vi "Xsens DeltaV (SubVI).vi"(1 "DATA in (Hex)":string) -> (0 "DeltaV":T1 {"DeltaVZ (m/s)" format="%#.7f"})   [LabVIEW 2019]
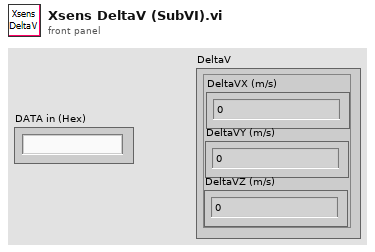
[diagram p1: front panel]
types:
  T1 = cluster{"DeltaVX (m/s)":sgl, "DeltaVY (m/s)":sgl, "DeltaVZ (m/s)":sgl}
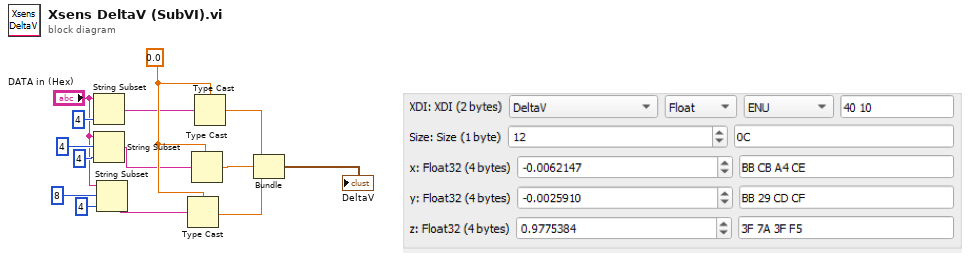
[diagram p0: block diagram]
diagram:
  w10 = sgl 0.0
  n1 = String Subset(string="DATA in (Hex)", length (rest)=4 ("length (rest)")) -> (substring=w8:string)  [unwired: 1 in]
  n2 = String Subset(string="DATA in (Hex)", offset (0)=4, length (rest)=4 ("length (rest)")) -> (substring=w3:string)
  n3 = String Subset(string="DATA in (Hex)", offset (0)=8, length (rest)=4 ("length (rest)")) -> (substring=w2:string)
  n4 = Type Cast(type=w10, x=w2) -> (*(type *) &x=w11:sgl)
  n5 = Type Cast(type=w10, x=w3) -> (*(type *) &x=w12:sgl)
  n6 = Type Cast(type=w10, x=w8) -> (*(type *) &x=w13:sgl)
  n7 = Bundle(w13, w12, w11) -> (→"DeltaV":cluster{sgl, sgl, sgl})  [unwired: 1 in]
